vi "Dequeue.vi"(0 "MessageQueue":refnum<queue>, 1 "EnqueueType (PreviewQueue)":T1, 5 "timeout in ms (-1)":i32=-1, 11 "error in (no error)":errorcluster) -> (4 "MessageQueue":refnum<queue>, 6 "Message":string, 8 "Message Data":variant, 10 "AcPwrBase":refnum<class "AcPwrBase.lvclass">, 15 "error out":errorcluster)   [LabVIEW 2018, in "AcPwrPlugins.lvlib"]
doc: "This VI removes an element from the queue. Each element is comprised of a message and data."
uses:
  AcPwrPlugins.lvlib
  clMessage.ctl
  AcPwrBaseClass/AcPwrBase.lvclass
  DequeueEnum.ctl
panel:
  out "timed out?":bool
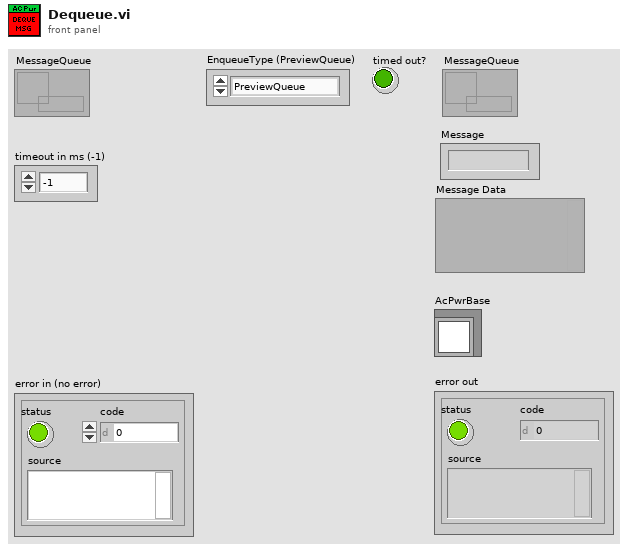
[diagram p1: front panel]
types:
  T1 = typedef "AcPwrPlugins.lvlib/DequeueEnum.ctl" = enum16{"PreviewQueue", "Dequeue"}
  T2 = typedef "AcPwrPlugins.lvlib/clMessage.ctl" = cluster{"Message":string, "Message Data":variant, "AcPwrBase":refnum<class "AcPwrBase.lvclass">}
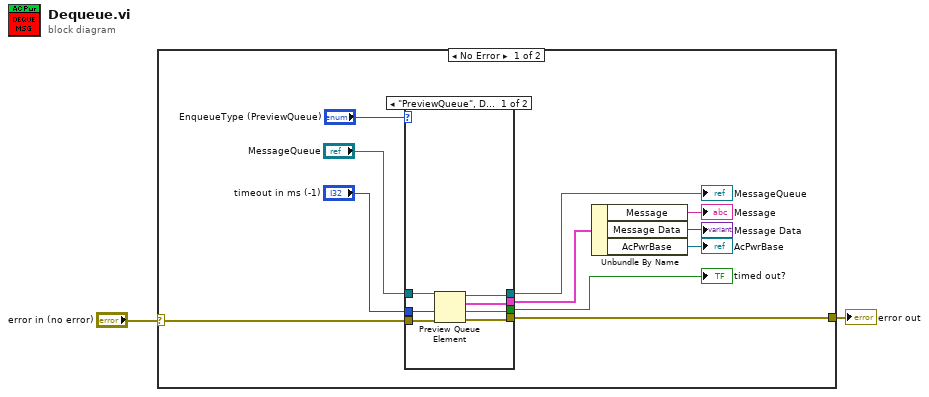
[diagram p0: block diagram]
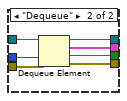
[diagram p2: hidden frame]
diagram:
  n1 = case shown="No Error" "error in (no error)" {
    selector: "error in (no error)" -> [w11 w28]
    tunnel: [w13 w28] -> w2
    frame No Error {
      n2 = case shown="\"PreviewQueue\", Default" "EnqueueType (PreviewQueue)" {
        tunnel: [w20 w27] -> w13
        tunnel: "MessageQueue" -> [w18 w26]
        tunnel: w11 -> [w19 w25]
        tunnel: [w16 w24] -> w10
        tunnel: [w17 w23] -> w7
        tunnel: "timeout in ms (-1)" -> [w15 w22]
        tunnel: [w14 w21] -> w5
        frame "PreviewQueue", Default {
          n3 = Preview Queue Element(queue=w18, timeout in ms (-1)=w15, error in (no error)=w19) -> (queue out=w17:refnum<queue>, element=w16:T2, timed out?=w14:bool, error out=w20:errorcluster)
        }
        frame "Dequeue" {
          n4 = Dequeue Element(queue=w26, timeout in ms (-1)=w22, error in (no error)=w25) -> (queue out=w23:refnum<queue>, element=w24:T2, timed out?=w21:bool, error out=w27:errorcluster)
        }
      }
      "MessageQueue" <- w7
      "timed out?" <- w5
      n5 = Unbundle By Name(w10) -> ("Message"=→"Message":string, "Message Data"=→"Message Data":variant, "AcPwrBase"=→"AcPwrBase":refnum<class "AcPwrBase.lvclass">)
    }
    frame Error {
    }
  }
  "error out" <- w2
